vi "Demo - Transfer Modes.vi"() -> ()   [LabVIEW 2020, in "GOLPI library.lvlib"]
doc: "Shows advantages and disadvantages of different transfer modes of data between GNU Octave and LabVIEW.\n\n---\nGOLPI works only with lv_proc.dll library, which is part of vipm package or should be delivered together with packed library. Placement of this dll is selected in terminal of Start GNU Octave.vi."
uses:
  GOLPI library.lvlib
  Private/Set Variable - polymorph parts/Set 1D Array Double.vi
  Private/Get Variable - polymorph parts/Get 1D Array Double.vi
  Private/Get Variable - polymorph parts/Get Struct.vi
panel:
  out "Pipe mode transfer time (s):":dbl[](array[numeric]) format="%#_3p"
  in  "stop":bool
  out "Bitstream mode transfer time (s):":dbl[](array[numeric]) format="%#_3p"
  out "Temporary file mode transfer time (s):":dbl[](array[numeric]) format="%#_3p"
  out "Normal mode transfer time (s):":dbl[](array[numeric]) format="%#_3p"
  in  "Test vector sizes":i32[](array[numeric])=[2, 20000]
  out "LabVIEW Cluster":T1
  in  "octave exe file or directory":path=path "C:/Octave/Octave-4.0.0/bin"
  out "exit code of GNU\nOctave process:":i32
  out "error out":errorcluster
  in  "working directory":path=path "C:/"
  # "1, start up"
  # "For Bitstream transsfer mode and for transfer of structures GNU Octave\npackage golpi is required. VIs will try to install it, if not found, you will be\nasked to find positiion of the fiel with the package.\n(golpi-X.X.X.tar.gz, where X is number)"
  # "GNU Octave is started, executable is placed in this directory:"
  # "Working directory is set to:"
  # "2, transfer mode speed comparison"
  # "Two vectors, small and large one, with number of elements                                          are prepared in LabVIEW."
  # "Normal tranfer mode: data are sent into GNU Octave using commands. Data are sent\nto LabVIEW  in such a way content of variables is printed to console and parsed by\nLabVIEW.\n\nTemporary file transfer mode: a temporary file in version 4 .mat format with the\ndata is created. Both GNU Octave and GOLPI can read the format directly.\n\nBitstream transfer mode: data are sent into GNU Octave using commands. Back to LabVIEW\ndata are converted into special series of bytes, bytes are printed to console and parsed\nby LabVIEW."
  # "These vectors are transfered to GNU Octave and back. Transfer times for different transfer modes are:"
  # "One can see the normal mode is fast for small data and slow for large ones. Using temporary file gives similar transfer \ntime, almost independent on the size of data. Bitstream mode gives faster results than normal mode, but output in \nconsole is not human readable."
  # "3, transfer of GNU Octave structure to LabVIEW cluster"
  # "GNU Octave structures can be transfered to LabVIEW cluster. Cluster must contain elements of the same name\nas structure fields and same data type. Structure can have extra fields and cluster can contain extra elements."
  # "In this example following structure is transfered to following cluster."
  # "GNU Octave structure\n\ns.num=5\ns.str=\"test\"\ns.mat = magic(3)\ns.not_in_cluster=-5"
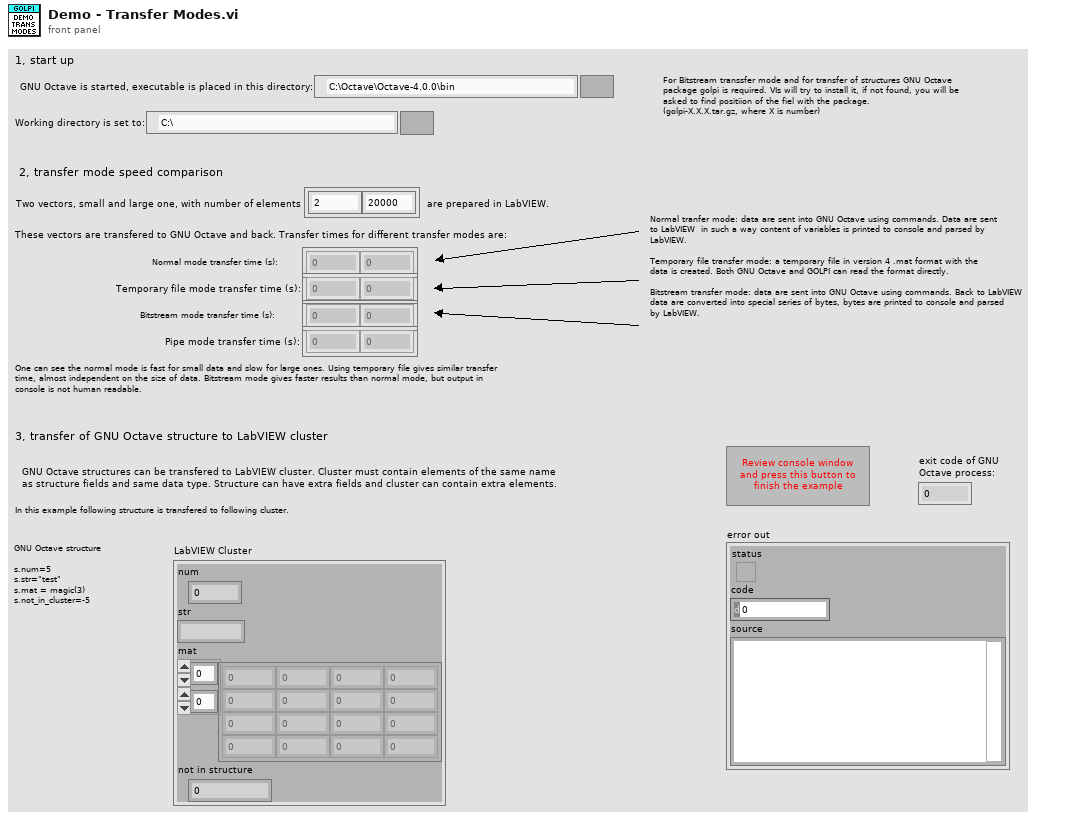
[diagram p1: front panel]
types:
  T1 = cluster{"num":dbl, "str":string, "mat":dbl[][], "not in structure":dbl}
  T2 = typedef "GOLPI library.lvlib/GOLPI reference Type Def.ctl" = cluster{"pipe handle":T3, "fast read timeout [ms]":u32, "fast read settle time [ms]":u32, "fast read to multiple [ms]":u32, "max elements per input line":u32, "slow read timeout [ms]":u32, "stdin double format specifier":string, "max elements per stdout output column":u32, "console mode bitstream":bool, "bitstream first read timeout [ms]":u32, "bitstream read timeout [ms]":u32, "struct transfer possible":bool, "matlab mode":bool, "var pipe write timeout [ms]":u32, "variable pipe mode":bool, "variable pipe buffer size [Bytes]":u32, "variable pipe block size [Bytes]":u32}
  T3 = typedef "LV Process library.lvlib/Pipe Handle.ctl" = cluster{"lv_proc.dll file path":path, "process instance handle":u32[], "debug mode":bool, "debug data":cluster{"time":timestamp, "stdin":bool, "data":string}[]}
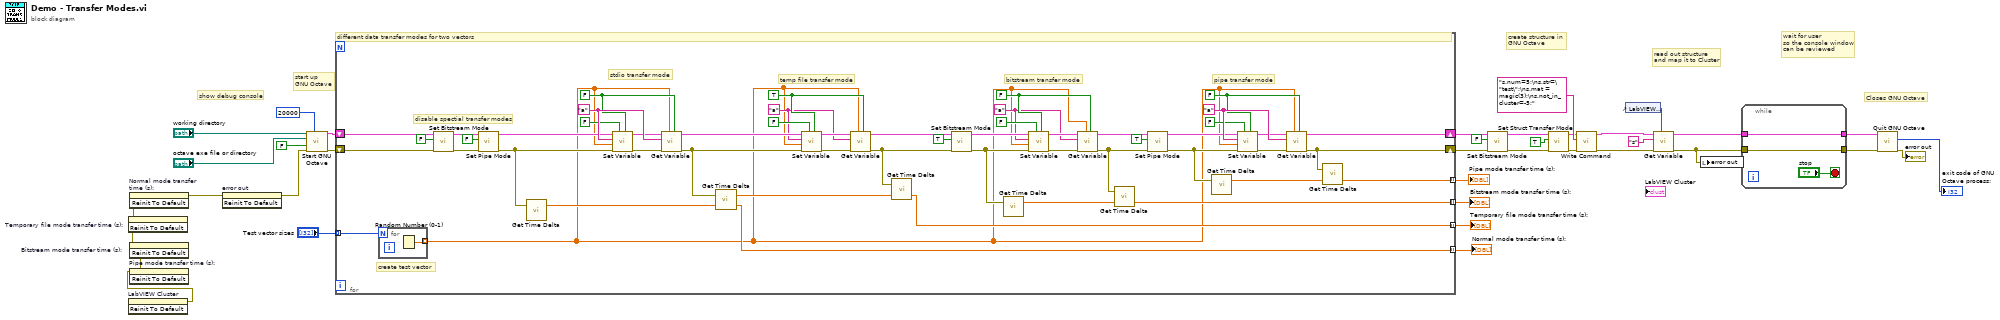
[diagram p0: block diagram]
diagram:
  # "wait for user\nso the console window\ncan be reviewed"
  # "read out structure\nand map it to Cluster"
  # "create structure in\nGNU Octave"
  # "start up\nGNU Octave"
  # "show debug console"
  # "Closes GNU Octave"
  n1 = invoke on="LabVIEW Cluster" class="Clust (strict)" method="Reinit To Default"() -> (error out=w1:errorcluster)  [unwired: 3 in, 2 out]
  n2 = invoke on="Pipe mode transfer time (s):" class="Arr (strict)" method="Reinit To Default"(error in=w1) -> (error out=w12:errorcluster)  [unwired: 2 in, 2 out]
  n3 = invoke on="Bitstream mode transfer time (s):" class="Arr (strict)" method="Reinit To Default"(error in=w12) -> (error out=w11:errorcluster)  [unwired: 2 in, 2 out]
  n4 = invoke on="Temporary file mode transfer time (s):" class="Arr (strict)" method="Reinit To Default"(error in=w11) -> (error out=w10:errorcluster)  [unwired: 2 in, 2 out]
  n5 = invoke on="Normal mode transfer time (s):" class="Arr (strict)" method="Reinit To Default"(error in=w10) -> (error out=w8:errorcluster)  [unwired: 2 in, 2 out]
  n6 = invoke on="error out" class="Clust (strict)" method="Reinit To Default"(error in=w8) -> (error out=w7:errorcluster)  [unwired: 2 in, 2 out]
  n7 = call "Start GNU Octave.vi"("working dir (user home)"="working directory", "full start timeout [ms] (20000)"=u32 20000 ("Full start timeout [ms] (5000)"), "octave binary file or dir (autofind)"="octave exe file or directory", "hide debug console (T)"=FALSE, "error in"=w7) -> ("GOLPI ref. out"=w30:T2, "error out"=w29:errorcluster)  [unwired: 7 in, 2 out]
  n8 = for {
    tunnel: "Test vector sizes" -> [w38] mode=indexing
    tunnel: [w77] -> w27 mode=indexing
    shift-right: [w40] -> w6
    shift-left: w29 -> [w84]
    shift-right: [w41] -> w3
    shift-left: w30 -> [w85]
    tunnel: [w76] -> w15 mode=indexing
    tunnel: [w75] -> w14 mode=indexing
    tunnel: [w39] -> w13 mode=indexing
    w49 = FALSE ("use temporary file? (F)")
    w52 = "a" ("variable name")
    w61 = FALSE ("use temporary file? (F)")
    w58 = "a" ("variable name")
    w67 = TRUE ("use temporary file? (F)")
    w64 = "a" ("variable name")
    w70 = FALSE ("use temporary file? (F)")
    w73 = "a" ("variable name")
    # "pipe transfer mode"
    # "bitstream transfer mode"
    # "temp file transfer mode"
    # "stdio transfer mode"
    # "disable spectial transfer modes"
    # "create test vector"
    # "different data transfer modes for two vectors"
    n9 = for {
      N: w38 -> [_]
      tunnel: [w89] -> w37 mode=indexing
      n10 = Random Number (0-1)() -> (number: 0 to 1=w89:dbl)
    }
    n11 = call "Set Bitstream Mode.vi"("error in"=w84, "Bitstream mode (F)"=FALSE, "GOLPI ref. in"=w85) -> ("error out"=w57:errorcluster, "GOLPI ref. out"=w55:T2)  [unwired: 7 in]
    n12 = call "Set Pipe Mode.vi"("error in"=w57, "Variable Pipe Mode? (F)"=FALSE, "GOLPI ref. in"=w55) -> ("error out"=w56:errorcluster, "GOLPI ref. out"=w54:T2)  [unwired: 7 in]
    n13 = call "Get Time Delta.vi"("anything in (for synchronization)"=w56) -> ("time now"=w82:dbl)  [unwired: 1 in, 1 out]
    n14 = call-poly "Set Variable.vi"("use temporary file? (F)"=w70, "column vector?"=FALSE, "error in"=w56, "value"=w37, "variable name"=w73, "GOLPI ref. in"=w54) -> ("error out"=w71:errorcluster, "GOLPI ref. out"=w72:T2)  [unwired: 4 in]
    n15 = call-poly "Get Variable.vi"("use temporary file? (F)"=w70, "data type of variable"=w37, "error in"=w71, "variable name"=w73, "GOLPI ref. in"=w72) -> ("error out"=w83:errorcluster, "GOLPI ref. out"=w88:T2)  [unwired: 4 in, 1 out]
    n16 = call "Get Time Delta.vi"("reference time (0)"=w82, "anything in (for synchronization)"=w83) -> ("time delta [s]"=w75:dbl, "time now"=w80:dbl)
    n17 = call-poly "Set Variable.vi"("use temporary file? (F)"=w67, "column vector?"=FALSE, "error in"=w83, "value"=w37, "variable name"=w64, "GOLPI ref. in"=w88) -> ("error out"=w66:errorcluster, "GOLPI ref. out"=w65:T2)  [unwired: 4 in]
    n18 = call-poly "Get Variable.vi"("use temporary file? (F)"=w67, "data type of variable"=w37, "error in"=w66, "variable name"=w64, "GOLPI ref. in"=w65) -> ("error out"=w81:errorcluster, "GOLPI ref. out"=w87:T2)  [unwired: 4 in, 1 out]
    n19 = call "Get Time Delta.vi"("reference time (0)"=w80, "anything in (for synchronization)"=w81) -> ("time delta [s]"=w76:dbl)  [unwired: 1 out]
    n20 = call "Set Bitstream Mode.vi"("error in"=w81, "Bitstream mode (F)"=TRUE, "GOLPI ref. in"=w87) -> ("error out"=w79:errorcluster, "GOLPI ref. out"=w86:T2)  [unwired: 7 in]
    n21 = call "Get Time Delta.vi"("anything in (for synchronization)"=w79) -> ("time now"=w78:dbl)  [unwired: 1 in, 1 out]
    n22 = call-poly "Set Variable.vi"("use temporary file? (F)"=w61, "column vector?"=FALSE, "error in"=w79, "value"=w37, "variable name"=w58, "GOLPI ref. in"=w86) -> ("error out"=w60:errorcluster, "GOLPI ref. out"=w59:T2)  [unwired: 4 in]
    n23 = call-poly "Get Variable.vi"("use temporary file? (F)"=w61, "data type of variable"=w37, "error in"=w60, "variable name"=w58, "GOLPI ref. in"=w59) -> ("error out"=w46:errorcluster, "GOLPI ref. out"=w43:T2)  [unwired: 4 in, 1 out]
    n24 = call "Get Time Delta.vi"("reference time (0)"=w78, "anything in (for synchronization)"=w46) -> ("time delta [s]"=w77:dbl)  [unwired: 1 out]
    n25 = call "Set Pipe Mode.vi"("error in"=w46, "Variable Pipe Mode? (F)"=TRUE, "GOLPI ref. in"=w43) -> ("error out"=w45:errorcluster, "GOLPI ref. out"=w44:T2)  [unwired: 7 in]
    n26 = call "Get Time Delta.vi"("anything in (for synchronization)"=w45) -> ("time now"=w47:dbl)  [unwired: 1 in, 1 out]
    n27 = call-poly "Set Variable.vi"("use temporary file? (F)"=w49, "column vector?"=FALSE, "error in"=w45, "value"=w37, "variable name"=w52, "GOLPI ref. in"=w44) -> ("error out"=w50:errorcluster, "GOLPI ref. out"=w51:T2)  [unwired: 4 in]
    n28 = call-poly "Get Variable.vi"("use temporary file? (F)"=w49, "data type of variable"=w37, "error in"=w50, "variable name"=w52, "GOLPI ref. in"=w51) -> ("error out"=w40:errorcluster, "GOLPI ref. out"=w41:T2)  [unwired: 4 in, 1 out]
    n29 = call "Get Time Delta.vi"("reference time (0)"=w47, "anything in (for synchronization)"=w40) -> ("time delta [s]"=w39:dbl)  [unwired: 1 out]
  }
  "Normal mode transfer time (s):" <- w14
  "Temporary file mode transfer time (s):" <- w15
  "Bitstream mode transfer time (s):" <- w27
  "Pipe mode transfer time (s):" <- w13
  n30 = call "Set Bitstream Mode.vi"("error in"=w6, "Bitstream mode (F)"=FALSE, "GOLPI ref. in"=w3) -> ("error out"=w5:errorcluster, "GOLPI ref. out"=w4:T2)  [unwired: 7 in]
  n31 = call "Set Struct Transfer Mode.vi"("error in"=w5, "Allow struct tranfer (False)"=TRUE, "GOLPI ref. in"=w4) -> ("error out"=w24:errorcluster, "GOLPI ref. out"=w25:T2)  [unwired: 6 in, 1 out]
  n32 = call "Write Command.vi"("error in"=w24, "command"="s.num=5;\ns.str=\"test\";\ns.mat = magic(3);\ns.not_in_cluster=-5;", "GOLPI ref. in"=w25) -> ("error out"=w22:errorcluster, "GOLPI ref. out"=w23:T2)  [unwired: 7 in]
  n33 = control-ref of="LabVIEW Cluster"() -> (w21:refnum<vi>)
  n34 = call-poly "Get Variable.vi"("cluster ref (empty)"=w21, "error in"=w22, "variable"="s", "GOLPI ref in"=w23) -> ("error out"=w9:errorcluster, "GOLPI ref. out"=w16:T2)  [unwired: 5 in, 1 out]
  n35 = local write "error out"(w9) -> ()
  n36 = while {
    tunnel: [w92] -> w18
    tunnel: w9 -> [w92]
    tunnel: [w90] -> w17
    tunnel: w16 -> [w90]
    stop <- "stop" stop-if-true
  }
  n37 = call "Quit GNU Octave.vi"("error in"=w18, "GOLPI ref. in"=w17) -> ("error out"=→"error out":errorcluster, "exit code"=→"exit code of GNU\nOctave process:":i32)  [unwired: 8 in]
